vi "Reply.vi"(7 "Sender":refnum<class "Sender.lvclass">, 9 "Priority?":bool, 10 "Msg Strategy":refnum<class "Msg Strategy.lvclass">, 11 "TEMPLATE jettl in":refnum<class "TEMPLATE jettl.lvclass">) -> (3 "TEMPLATE jettl out":refnum<class "TEMPLATE jettl.lvclass">)   [LabVIEW 2021, in "_Template.lvlib" / "Templates.lvlib" / "TEMPLATE jettl.lvlib" / "TEMPLATE jettl.lvclass"]
uses:
  TEMPLATE jettl.lvclass
  jettl/jettl/Sender/Sender/Sender.lvclass
  jettl/jettl/Msg Strategy/Msg Strategy.lvclass
  TEMPLATE jettl.lvclass/TEMPLATE jettl.ctl
  jettl/jettl/jettl/jettl.lvclass
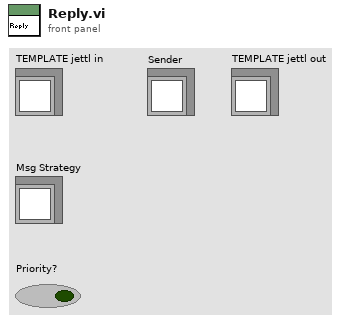
[diagram p1: front panel]
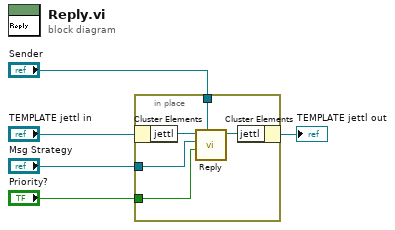
[diagram p0: block diagram]
diagram:
  n1 = in-place {
    in-place-border: "Sender" -> [w8]
    in-place-border: "Msg Strategy" -> [w7]
    in-place-border: "Priority?" -> [w6]
    n2 = in-place-cluster #1("TEMPLATE jettl in") -> ("jettl"=w10:refnum<class "jettl.lvclass">)
    n3 = call-dynamic "Reply.vi"("Sender"=w8, "Priority?"=w6, "Msg Strategy"=w7, "jettl in"=w10) -> ("jettl out"=w9:refnum<class "jettl.lvclass">)  [unwired: 7 in]
    n4 = in-place-cluster #1("jettl"=w9) -> (→"TEMPLATE jettl out":refnum<class "TEMPLATE jettl.lvclass">)
  }
